vi "fibonacci.vi"(9 "n":u8, 11 "cache in":i32[](array[numeric])) -> (1 "F(n)":i32, 3 "cache out":i32[](array[numeric]))   [LabVIEW 2021]
doc: "程序的说明请查看我的bl og： \nhttp://ruanqizhen.spaces.live.com/blog/cns!5852D4F797C53FB6!1832.entry"
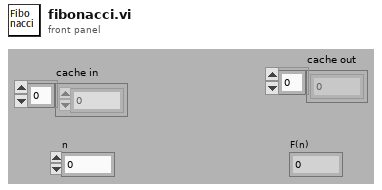
[diagram p1: front panel]
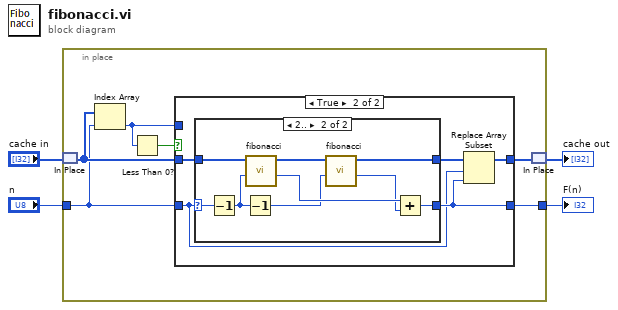
[diagram p0: block diagram]
diagram:
  n1 = in-place {
    in-place-border: [w9] -> w4
    in-place-border: "n" -> [w5]
    n2 = in-place-match #1("cache in") -> (w8:i32[])
    n3 = Index Array(array=w8, index=w5) -> (element=w6:i32)
    n4 = Less Than 0?(x=w6) -> (x < 0?=w10:bool)
    n5 = case shown="True" w10 {
      tunnel: [w11 w16] -> w9
      tunnel: w5 -> [_ w15]
      tunnel: w8 -> [w12 w17]
      tunnel: [w12 w13] -> w7
      tunnel: w6 -> [w11 _]
      frame False {
      }
      frame True {
        n6 = case shown="2.." w15 {
          selector: w15 -> [w19 w28]
          tunnel: [w19 w27] -> w16
          tunnel: w17 -> [w18 w22]
          tunnel: [w18 w21] -> w14
          frame ..1, Default {
          }
          frame 2.. {
            n7 = Decrement(x=w28) -> (x-1=w20:u8)
            n8 = Decrement(x=w20) -> (x-1=w25:u8)
            n9 = call "fibonacci.vi"("n"=w20, "cache in"=w22) -> ("F(n)"=w26:i32, "cache out"=w23:i32[])  [unwired: 8 in]
            n10 = call "fibonacci.vi"("n"=w25, "cache in"=w23) -> ("F(n)"=w24:i32, "cache out"=w21:i32[])  [unwired: 8 in]
            n11 = Add(x=w26, y=w24) -> (x+y=w27:i32)
          }
        }
        n12 = Replace Array Subset(array=w14, new element=w16, index=w15) -> (w13:i32[])
      }
    }
    n13 = in-place-match #1(w7) -> (→"cache out":i32[])
  }
  "F(n)" <- w4
